vi "get_current_set_low_limit.vi"(8 "error in":errorcluster, 11 "VISA resource name":refnum<visa-resource-name>="COM1") -> (0 "error out":errorcluster, 3 "Response":string)   [LabVIEW 2020]
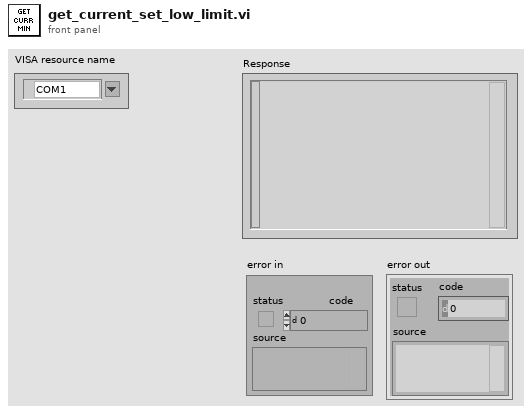
[diagram p1: front panel]
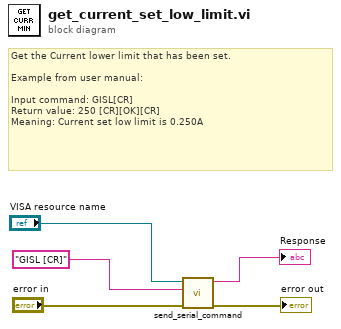
[diagram p0: block diagram]
diagram:
  # "Get the Current lower limit that has been set.\n\nExample from user manual:\n\nInput command: GISL[CR]\nReturn value: 250 [CR][OK][CR]\nMeaning: Current set low limit is 0.250A"
  n1 = call "send_serial_command.vi"("error in (no error)"="error in", "Command"="GISL [CR]", "VISA resource name"="VISA resource name") -> ("error out"=→"error out":errorcluster, "Response"=→"Response":string)  [unwired: 7 in]
